vi "create Timings.vi"(8 "error in (no error)":errorcluster, 10 "Parameters":u32[](array[numeric]), 11 "ESD in":refnum<class "ESD.lvclass">) -> (0 "error out":errorcluster, 1 "wait":i32[](array[numeric])=[0, 30000, 0, 0], 2 "timeout":u32[](array[numeric]), 3 "ESD out":refnum<class "ESD.lvclass">)   [LabVIEW 2013, in "ESD.lvclass"]
uses:
  ESD.lvclass
  TestInterface/TestInterface.lvclass
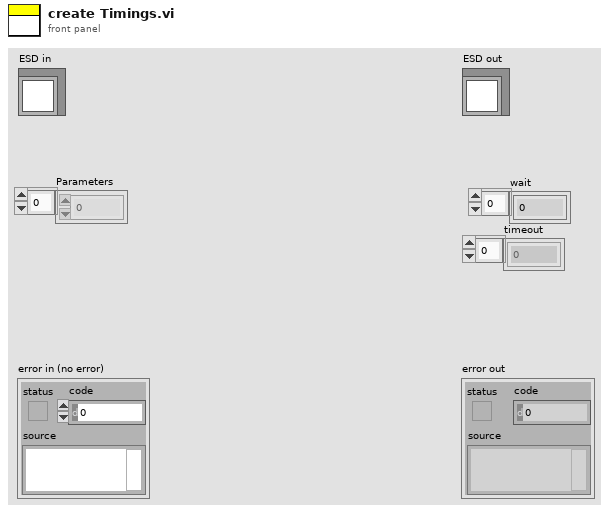
[diagram p1: front panel]
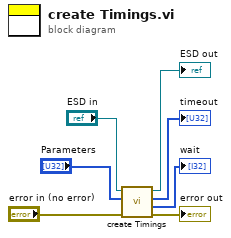
[diagram p0: block diagram]
diagram:
  n1 = call-parent "create Timings.vi"("error in (no error)"="error in (no error)", "Parameters"="Parameters", "TestInterface in"="ESD in") -> ("error out"=→"error out":errorcluster, "wait"=→"wait":i32[], "timeout"=→"timeout":u32[], "TestInterface out"=→"ESD out":refnum<class "ESD.lvclass">)  [unwired: 5 in]
